vi "FTW-Socket-Subscribe.vi"(0 "FTW Socket":refnum<class "FTW-Socket.lvclass">, 5 "Topic":string, 11 "error in":errorcluster) -> (4 "FTW Socket out":refnum<class "FTW-Socket.lvclass">, 15 "error out":errorcluster)   [LabVIEW 2013, in "FTW-Socket.lvclass"]
uses:
  FTW-Socket.lvclass
  FTW-Socket.lvclass/FTW-Socket.ctl
  error/FTW-ERR-ThrowGenericError.vi
  error/FTW-ERR-ThrowError.vi
  error/FTW-ERR-NoErrorConstant.vi
  error/FTW-ERR-CallChain.vi
  string/FTW-STR-ReplaceWhitespace.vi
panel:
  # "Inputs"
  # "Outputs"
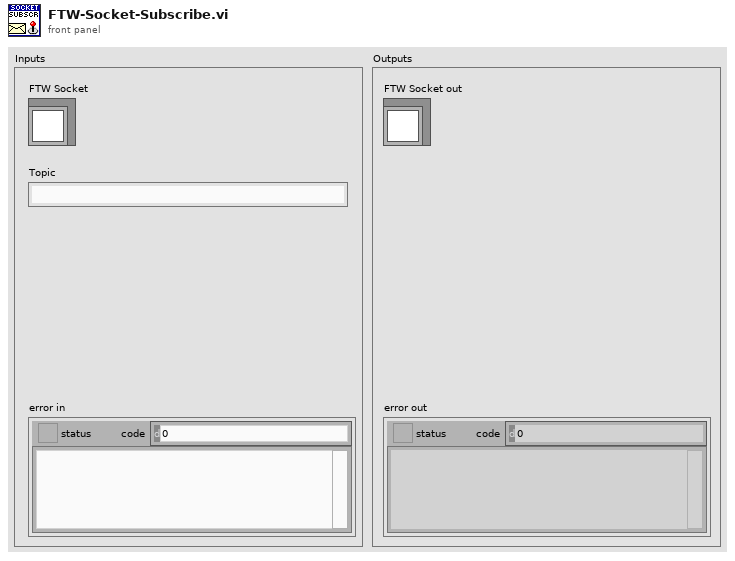
[diagram p1: front panel]
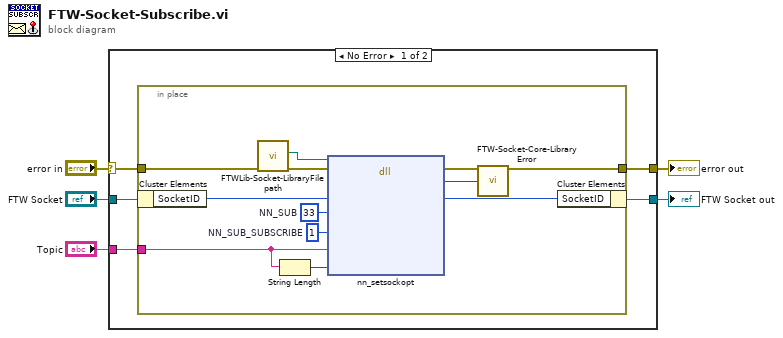
[diagram p0: block diagram]
diagram:
  n1 = case shown="No Error" "error in" {
    selector: "error in" -> [w8 w23]
    tunnel: "FTW Socket" -> [w10 w24]
    tunnel: [w6 w23] -> w4
    tunnel: [w9 w24] -> w3
    tunnel: "Topic" -> [w7 _]
    frame No Error {
      n2 = in-place {
        in-place-border: w8 -> [w21]
        in-place-border: [w16] -> w6
        in-place-border: w7 -> [w14]
        w11 = 33  # NN_SUB
        w12 = 1  # NN_SUB_SUBSCRIBE
        n3 = in-place-cluster #1(w10) -> ("SocketID"=w22:i64)
        n4 = call "FTWLib-Socket-LibraryFilepath.vi"("error in"=w21) -> ("error out"=w19:errorcluster, "Library Filepath"=w18:path)  [unwired: 8 in, 1 out]
        n5 = String Length(string=w14) -> (length=w13:i32)
        n6 = dll-call lib="C:/Users/Jack/repo/ftw-vps/ftw/lib/nanomsg/FTWLib-nanomsg32.dll" fn="nn_setsockopt"(path in=w18, error in=w19, "SocketID"=w22, "Level"=w11, "Option"=w12, "Value"=w14, "Length"=w13) -> (error out=w17:errorcluster, "Return Value"=w15:i64, "SocketID"=w20:i64)  [unwired: 5 in, 1 out]
        n7 = call "FTW-Socket-Core-LibraryError.vi"("error in"=w17, "Return Value"=w15) -> ("error out"=w16:errorcluster)  [unwired: 13 in]
        n8 = in-place-cluster #1("SocketID"=w20) -> (w9:refnum<class "FTW-Socket.lvclass">)
      }
    }
    frame Error {
    }
  }
  "error out" <- w4
  "FTW Socket out" <- w3
